vi "_FPGA Write I32 Array.vi"(4 "error in":errorcluster, 5 "U32 Array":u32[](array[numeric]), 6 "Offset (0)":u16) -> (0 "error out":errorcluster, 2 "Next Offset":u16)   [LabVIEW 2015]
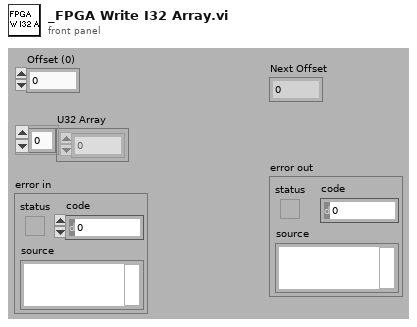
[diagram p1: front panel]
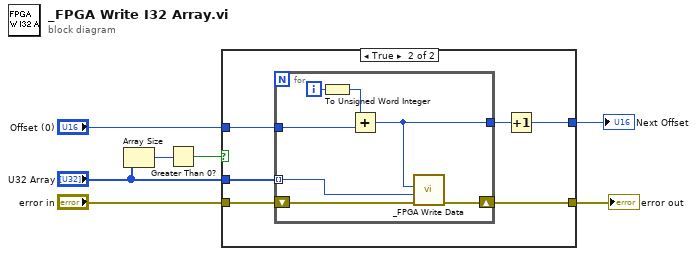
[diagram p0: block diagram]
diagram:
  n1 = Array Size(array="U32 Array") -> (size(s)=w4:i32)
  n2 = Greater Than 0?(x=w4) -> (x > 0?=w5:bool)
  n3 = case shown="True" w5 {
    tunnel: "Offset (0)" -> [w9 w15]
    tunnel: "U32 Array" -> [_ w14]
    tunnel: [w9 w12] -> w3
    tunnel: "error in" -> [w8 w11]
    tunnel: [w8 w10] -> w1
    frame False {
    }
    frame True {
      n4 = for {
        shift-right: [w21] -> w10
        shift-left: w11 -> [w22]
        tunnel: w14 -> [w20] mode=indexing
        tunnel: w15 -> [w19]
        tunnel: [w18] -> w13
        i -> [w17]
        n5 = To Unsigned Word Integer(number=w17) -> (unsigned 16bit integer=w16:u16)
        n6 = Add(x=w16, y=w19) -> (x+y=w18:u16)
        n7 = call "_FPGA Write Data.vi"("error in"=w22, "Data"=w20, "Address"=w18) -> ("error out"=w21:errorcluster)  [unwired: 3 in, 2 out]
      }
      n8 = Increment(x=w13) -> (x+1=w12:u16)
    }
  }
  "Next Offset" <- w3
  "error out" <- w1
